vi "Send GetTaskStatus.vi"(7 "Message Priority (Normal)":T6=enum."Normal", 8 "error in (no error)":errorcluster, 11 "Message Enqueuer":refnum<class "Message Enqueuer.lvclass">) -> (0 "error out":errorcluster, 2 "TaskStatus":T5 {"Acessors:TaskConfig"."SampleRateConfiguration"."SampleMode" items=["Finite Samples"=10178, "Continuous Samples"=10123, "Hardware Timed Single Point"=12522]}, 3 "Message Enqueuer out":refnum<class "Message Enqueuer.lvclass">)   [LabVIEW 2025, in "Task_Abstr.lvlib" / "GetTaskStatus Msg.lvclass"]
doc: "This VI sends the message to an actor."
uses:
  GetTaskStatus Msg.lvclass
  <vilib>/ActorFramework/Message Enqueuer/Message Enqueuer.lvclass
  <vilib>/ActorFramework/Message Enqueuer/Message Priority.ctl
  DAQ_Module/DAQ_Module/DAQ_Module/DAQ_Task_Config.ctl
  DAQ_Module/DAQ_Module/DAQ_Module/DAQ_HW_Type.ctl
  DAQ_Module/DAQ_Module/DAQ_Module/DAQ_Task_Type.ctl
  DAQ_Module/DAQ_Module/DAQ_Module/DAQ_SampleRateConfig.ctl
  C:/Program Files (x86)/National Instruments/LabVIEW 2025/vi.lib/ActorFramework/Message/Message.lvclass
  GetTaskStatus Msg.lvclass/GetTaskStatus Msg.ctl
  <vilib>/ActorFramework/Message Enqueuer/Message Enqueuer.lvclass/Message Enqueuer.ctl
  <vilib>/ActorFramework/Message Priority Queue/Priority Enqueue.vi
  DAQ_Module/DAQ_Module/DAQ_Module/DAQ_Module.lvclass
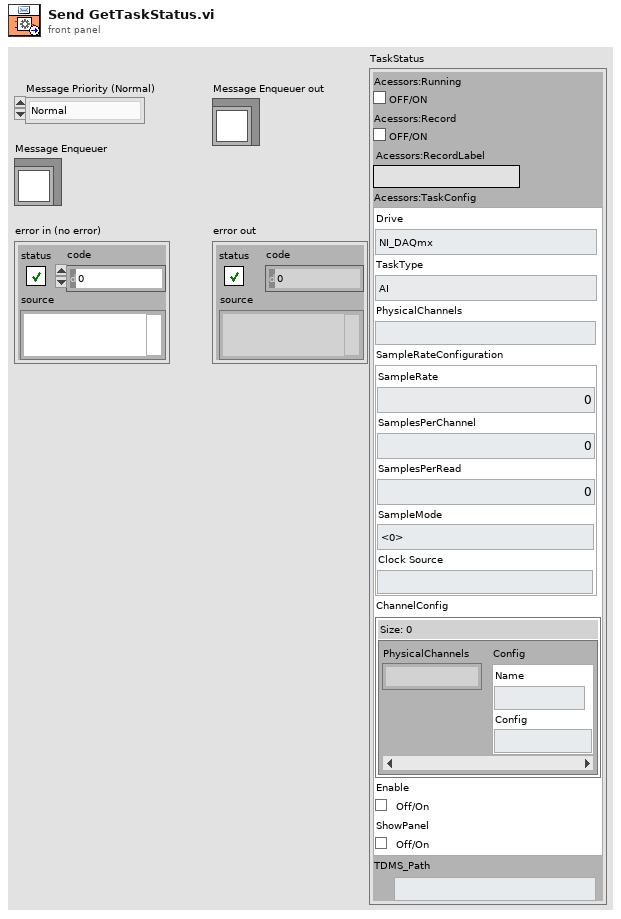
[diagram p1: front panel]
types:
  T1 = typedef "DAQ_Module.lvlib/DAQ_Module.lvclass/DAQ_Task_Config.ctl" = cluster{"Drive":T2, "TaskType":T3, "PhysicalChannels":string, "SampleRateConfiguration":T4, "ChannelConfig":map{string, cluster{"Name":string, "Config":string}}, "Enable":bool, "ShowPanel":bool}
  T2 = typedef "DAQ_Module.lvlib/DAQ_Module.lvclass/DAQ_HW_Type.ctl" = enum16{"NI_DAQmx", "Simulated_DAQ"}
  T3 = typedef "DAQ_Module.lvlib/DAQ_Module.lvclass/DAQ_Task_Type.ctl" = enum16{"AI", "Linear", "Angular", "AO"}
  T4 = typedef "DAQ_Module.lvlib/DAQ_Module.lvclass/DAQ_SampleRateConfig.ctl" = cluster{"SampleRate":dbl, "SamplesPerChannel":u32, "SamplesPerRead":i32, "SampleMode":i32, "Clock Source":string}
  T5 = cluster{"Acessors:Running":bool, "Acessors:Record":bool, "Acessors:RecordLabel":string, "Acessors:TaskConfig":T1, "TDMS_Path":path}
  T6 = typedef "Actor Framework.lvlib/Message Enqueuer.lvclass/Message Priority.ctl" = enum16{"Low", "Normal", "High"}
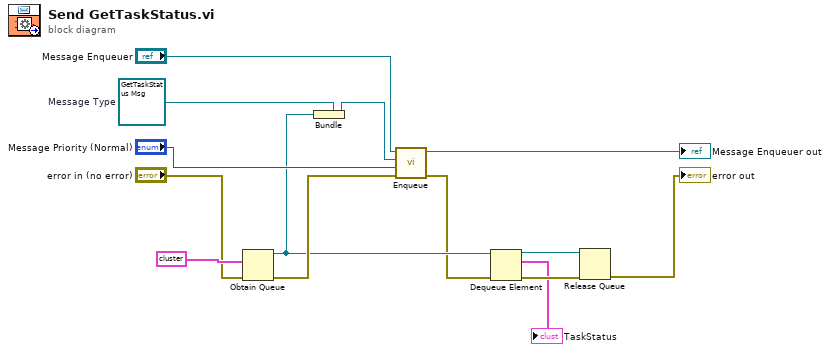
[diagram p0: block diagram]
diagram:
  w13 = refnum<class "GetTaskStatus Msg.lvclass"> refnum  # Message Type
  n1 = Obtain Queue(element data type=T5 {"Acessors:Running"=FALSE, "Acessors:Record"=FALSE, "Acessors:RecordLabel"="", "Acessors:TaskConfig"={"Drive"=enum."NI_DAQmx", "TaskType"=enum."AI", "PhysicalChannels"="", "SampleRateConfiguration"={"SampleRate"=0.0, "SamplesPerChannel"=0, "SamplesPerRead"=0, "SampleMode"=0, "Clock Source"=""}, "ChannelConfig"={}, "Enable"=FALSE, "ShowPanel"=FALSE}, "TDMS_Path"=path ""} ("TaskStatus"), error in (no error)="error in (no error)") -> (queue out=w6:refnum<queue>, error out=w7:errorcluster)  [unwired: 3 in, 1 out]
  n2 = Bundle(cluster=w13, w6) -> (w9:refnum<class "GetTaskStatus Msg.lvclass">)
  n3 = call <vilib>:"Enqueue.vi"("error in (no error)"=w7, "Message Priority (Normal)"="Message Priority (Normal)", "Message"=w9, "Message Enqueuer in"="Message Enqueuer") -> ("error out"=w5:errorcluster, "Message Enqueuer out"=→"Message Enqueuer out":refnum<class "Message Enqueuer.lvclass">)  [unwired: 6 in]
  n4 = Dequeue Element(queue=w6, error in (no error)=w5) -> (queue out=w4:refnum<queue>, element=→"TaskStatus":T5, error out=w3:errorcluster)  [unwired: 1 in, 1 out]
  n5 = Release Queue(queue=w4, error in (no error)=w3) -> (error out=→"error out":errorcluster)  [unwired: 1 in, 2 out]
